vi "RWNoise-Averager.vi"(0 "RW Noise Params":T28, 5 "Runtime":T2={"Stimulus"={"Waveform"={"Type"=enum."Tone", "Tone"={"Frequency (kHz)"=0.0, "Last Freq"=0.0, "Last Phase"=0.0}, "Pulse Train"={"Pulse width (us)"=0.0, "Pulse rate (Hz)"=0.0, "Gap (ms)"=0.0, "Polarity"=enum."POS", "PT State"={"Template"=[], "Nperiod"=0, "Index"=0, "Pulse Rate (Hz)"=0.0, "Phase (cycles)"=0.0, "Noff"=0}, "Asynch"=FALSE}, "Noise"={"InvFilt"=FALSE, "Noise"=[], "CurPt"=0, "Aweight"=FALSE, "Seed"=0, "afile"=path ""}, "File"={"Filename"=path "", "Signal"=[], "Channel"=0, "stream"=FALSE, "offset"=0, "nreps"=0, "loops"=0, "Randomize"=FALSE, "order"=[], "Seed"=0, "Tokens"=0}, "FMSweep"={"Rate (oct/s)"=0.0, "Fmin (Hz)"=0.0, "Fmax (Hz)"=0.0, "Ramp (ms)"=0.0, "Linear"=FALSE}, "Chirp Train"={"Params"={"Fmin (kHz)"=4.0, "Fmax (kHz)"=64.0, "Compensate"=FALSE, "Duration (ms)"=2.0}, "Data"={"WF"=[]}}, "Complex Tone"={"Params"={"F0 (Hz)"=0.0, "Band"={"Flow (Hz)"=0.0, "Fhigh (Hz)"=0.0}, "Phase"=enum."Cosine", "Min F0 (Hz)"=0.0, "Max F0 (Hz)"=0.0, "ContinRandPhase"=FALSE, "Max peak factor"=inf, "Max mod depth"=2.0, "MinHarmNum"=0, "MaxHarmNum"=0, "Level Mode"=enum."per component", "% jitter"=0.0}, "Data"={"Ncomp"=0, "MinHarm"=0, "Phase"=[], "Amplitude"=[], "Npts/frame"=0, "Last F0"=0.0, "Fmin"=0.0, "Fmax"=0.0, "Lslope"=0.0, "randphase"=FALSE, "overall rms"=FALSE, "fmult"=[], "jittered"=FALSE}}, "Moving Ripple"={"Params"={"Fmin"=0.0, "Fmax"=0.0, "Density"=0.0, "Velocity"=0.0, "Depth"=0.0, "Phase"=0.0, "Comp/oct"=0}, "Data"={"Freq"=[], "A"=[], "phase"=[], "Phase"=0.0}}}, "Filter"={"Type"=enum."Lowpass", "CF (kHz)"=0.0, "BW (kHz)"=0.0, "Cascade"=FALSE, "Quadrature"=FALSE, "Scale Factor"=0.0, "Stages"=[], "Class"=enum."Elliptic", "Order"=0, "BWUnits"=enum."Linear"}, "Burst"={"Active"=FALSE, "Delay (ms)"=0.0, "Duration (ms)"=0.0, "Ramp (ms)"=0.0, "Rate (Hz)"=0.0, "Trepeat (ms)"=0.0, "Repeat"=FALSE}, "Level"={"Level"=0.0, "Units"=enum."dB atten", "Max"=0.0, "Multiplier"=0.0, "Cal File"=path "", "Cal"={"Freq (Hz)"=[], "Mag (dB SPL)"=[], "Phase (deg)"=[]}}, "Name"="", "Advanced"={"Rep Mask"="", "AltPol"=FALSE, "Var"="", "Expr"="", "Persist"=FALSE}, "SAM"={"Active"=FALSE, "Frequency (Hz)"=0.0, "Depth"=0.0, "Init Phase (cycles)"=0.0, "phase (degrees)"=0.0, "Asynch"=FALSE}}, "Fs (Hz)"=0.0, "AO Npts"=0, "AO Channels"=[], "Active"=FALSE, "AINpts"=0, "WinPts"=0, "NUpdate"=0} {"Stimulus"."Filter"."Stages"."IIR Filter"."Forward Coefficients" format="%.4f"; "Stimulus"."Filter"."Stages"."IIR Filter"."Reverse Coefficients" format="%.4f"}, 11 "error in (no error)":errorcluster, 12 "Refs":T1) -> (8 "Spectrum (uV)":dbl[](array[numeric]), 15 "error out":errorcluster)   [LabVIEW 2020]
uses:
  RWNoise Params.ctl
  epl-vi-lib/Utility VIs/Type Defs/Left-Right ring.ctl
  RWNoise-Runtime Data.ctl
  epl-vi-lib/Signal Synthesis VIs/Controls/Stimulus Channel (Full)/Full Stimulus Channel Data.ctl
  epl-vi-lib/Signal Synthesis VIs/Controls/Waveform XCtl/Waveform Data.ctl
  epl-vi-lib/Signal Synthesis VIs/Controls/Waveform XCtl/Waveform Enum.ctl
  epl-vi-lib/Signal Synthesis VIs/Waveform VIs/Tone VIs/Tone Params.ctl
  epl-vi-lib/Signal Synthesis VIs/Waveform VIs/Pulse Train VIs/Pulse Train Params.ctl
  epl-vi-lib/Signal Synthesis VIs/Waveform VIs/Pulse Train VIs/Pulse Polarity.ctl
  epl-vi-lib/Signal Synthesis VIs/Waveform VIs/Pulse Train VIs/PT-Continuous State.ctl
  epl-vi-lib/Signal Synthesis VIs/Waveform VIs/Noise VIs/Noise Params.ctl
  epl-vi-lib/Signal Synthesis VIs/Waveform VIs/File VIs/StimFile-Params.ctl
  epl-vi-lib/Signal Synthesis VIs/Waveform VIs/FM Sweep VIs/FM Sweep Params.ctl
  epl-vi-lib/Signal Synthesis VIs/Waveform VIs/Chirp Train VIs/Chirp Train.ctl
  epl-vi-lib/Signal Synthesis VIs/Waveform VIs/Chirp Train VIs/Chirp Train Params.ctl
  epl-vi-lib/Signal Synthesis VIs/Waveform VIs/Complex Tone VIs/CT-Params.ctl
  epl-vi-lib/Signal Synthesis VIs/Waveform VIs/Complex Tone VIs/CT-Phase Enum.ctl
  epl-vi-lib/Signal Synthesis VIs/Waveform VIs/Complex Tone VIs/CT-Runtime Data.ctl
  epl-vi-lib/Signal Synthesis VIs/Waveform VIs/Moving Ripple VIs/Moving Ripple.ctl
  epl-vi-lib/Signal Synthesis VIs/Waveform VIs/Moving Ripple VIs/Moving Ripple.Params.ctl
  epl-vi-lib/Signal Synthesis VIs/Waveform VIs/Moving Ripple VIs/Moving Ripple.Data.ctl
  epl-vi-lib/Signal Synthesis VIs/Controls/Advanced Filter XCtl/Filter Data.ctl
  epl-vi-lib/Signal Synthesis VIs/Filter VIs/Filter-Bandwidth Units.ctl
  epl-vi-lib/Signal Synthesis VIs/Controls/Burst XCtl/Burst Data.ctl
  epl-vi-lib/Signal Synthesis VIs/Controls/Level XCtl/Level Data.ctl
  epl-vi-lib/Signal Synthesis VIs/Controls/Level XCtl/Level Units.ctl
  epl-vi-lib/Signal Synthesis VIs/Controls/Advanced Options XCtl/Advanced Stimulus Options.ctl
  epl-vi-lib/Signal Synthesis VIs/Modulation VIs/SAM VIs/SAM Params.ctl
  RWNoise-Control Refs.ctl
  <vilib>/Analysis/4window.llb/Hanning Window (DBL).vi
  <vilib>/Analysis/4window.llb/AllCosWindow (DBL).vi
  <vilib>/Analysis/NI_AALPro.lvlib
  epl-vi-lib/Signal Synthesis VIs/Controls/Advanced Filter XCtl/Advanced Filter XCtl.xctl
  epl-vi-lib/Signal Synthesis VIs/Controls/Level XCtl/Level XCtl.xctl
  epl-vi-lib/Signal Synthesis VIs/Controls/Burst XCtl/Burst Control.xctl
  epl-vi-lib/Signal Synthesis VIs/Controls/Waveform XCtl/Waveform XCtl.xctl
  epl-vi-lib/Signal Synthesis VIs/Controls/Advanced Options XCtl/Advanced Stimulus Options.xctl
  epl-vi-lib/Signal Synthesis VIs/Controls/Stimulus Channel (Full)/Stimulus Channel (Full).xctl
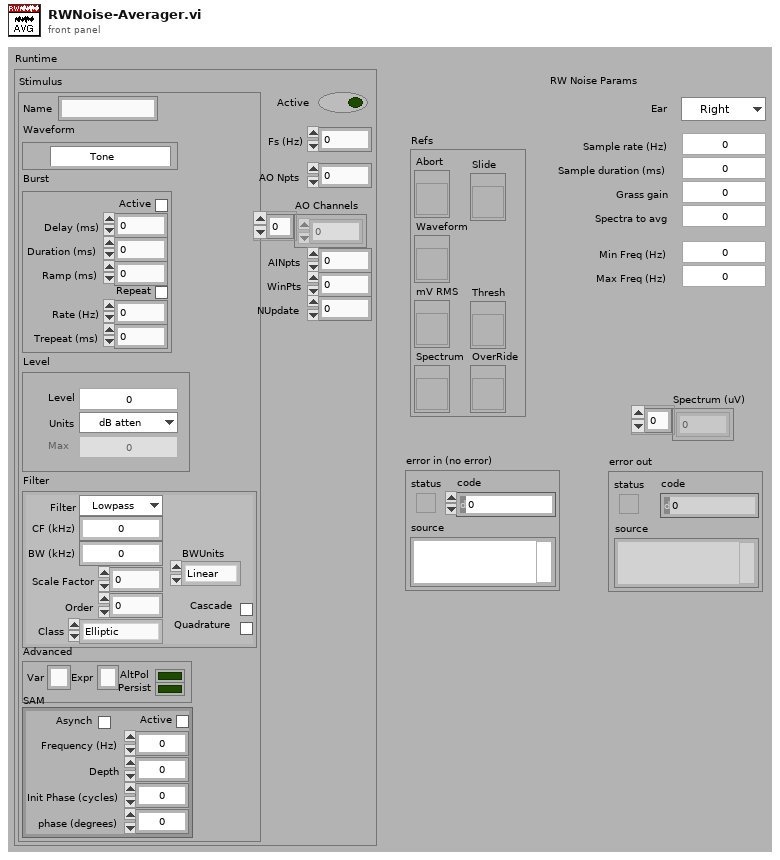
[diagram p1: front panel]
types:
  T1 = typedef "RWNoise-Control Refs.ctl" = cluster{"Abort":refnum<vi>, "Waveform":refnum<vi>, "mV RMS":refnum<vi>, "Spectrum":refnum<vi>, "Slide":refnum<vi>, "Thresh ":refnum<vi>, "OverRide":refnum<vi>}
  T2 = typedef "RWNoise-Runtime Data.ctl" = cluster{"Stimulus":T3, "Fs (Hz)":dbl, "AO Npts":i32, "AO Channels":i32[], "Active":bool, "AINpts":i32, "WinPts":i32, "NUpdate":i32}
  T3 = typedef "Stimulus Channel (Full).xctl/Full Stimulus Channel Data.ctl" = cluster{"Waveform":T4, "Filter":T21, "Burst":T23, "Level":T24, "Name":string, "Advanced":T26, "SAM":T27}
  T4 = typedef "Waveform XCtl.xctl/Waveform Data.ctl" = cluster{"Type":T5, "Tone":T6, "Pulse Train":T7, "Noise":T10, "File":T11, "FMSweep":T12, "Chirp Train":T13, "Complex Tone":cluster{"Params":T15, "Data":T17}, "Moving Ripple":T18}
  T5 = typedef "Waveform Enum.ctl" = enum16{"OFF", "Tone", "Noise", "Pulse Train", "File", "FM Sweep", "Chirp Train", "Complex Tone", "FM Tone", "Moving Ripple"}
  T6 = typedef "Tone Params.ctl" = cluster{"Frequency (kHz)":dbl, "Last Freq":dbl, "Last Phase":dbl}
  T7 = typedef "Pulse Train Params.ctl" = cluster{"Pulse width (us)":dbl, "Pulse rate (Hz)":dbl, "Gap (ms)":dbl, "Polarity":T8, "PT State":T9, "Asynch":bool}
  T8 = typedef "Pulse Polarity.ctl" = enum16{"POS", "NEG", "POS-NEG", "NEG-POS"}
  T9 = typedef "PT-Continuous State.ctl" = cluster{"Template":dbl[], "Nperiod":i32, "Index":i32, "Pulse Rate (Hz)":dbl, "Phase (cycles)":dbl, "Noff":i32}
  T10 = typedef "Noise Params.ctl" = cluster{"InvFilt":bool, "Noise":dbl[], "CurPt":i32, "Aweight":bool, "Seed":i32, "afile":path}
  T11 = typedef "StimFile-Params.ctl" = cluster{"Filename":path, "Signal":dbl[], "Channel":i32, "stream":bool, "offset":i32, "nreps":i32, "loops":i32, "Randomize":bool, "order":i32[], "Seed":i32, "Tokens":i32}
  T12 = typedef "FM Sweep Params.ctl" = cluster{"Rate (oct/s)":dbl, "Fmin (Hz)":dbl, "Fmax (Hz)":dbl, "Ramp (ms)":dbl, "Linear":bool}
  T13 = typedef "Chirp Train.ctl" = cluster{"Params":T14, "Data":cluster{"WF":dbl[]}}
  T14 = typedef "Chirp Train Params.ctl" = cluster{"Fmin (kHz)":dbl, "Fmax (kHz)":dbl, "Compensate":bool, "Duration (ms)":dbl}
  T15 = typedef "CT-Params.ctl" = cluster{"F0 (Hz)":dbl, "Band":cluster{"Flow (Hz)":dbl, "Fhigh (Hz)":dbl}, "Phase":T16, "Min F0 (Hz)":dbl, "Max F0 (Hz)":dbl, "ContinRandPhase":bool, "Max peak factor":dbl, "Max mod depth":dbl, "MinHarmNum":i32, "MaxHarmNum":i32, "Level Mode":enum16{"per component", "overall rms"}, "% jitter":dbl}
  T16 = typedef "CT-Phase Enum.ctl" = enum16{"Cosine", "Random", "Alternating"}
  T17 = typedef "CT-Runtime Data.ctl" = cluster{"Ncomp":i32, "MinHarm":i32, "Phase":dbl[], "Amplitude":dbl[], "Npts/frame":i32, "Last F0":dbl, "Fmin":dbl, "Fmax":dbl, "Lslope":dbl, "randphase":bool, "overall rms":bool, "fmult":dbl[], "jittered":bool}
  T18 = typedef "Moving Ripple.ctl" = cluster{"Params":T19, "Data":T20}
  T19 = typedef "Moving Ripple.Params.ctl" = cluster{"Fmin":dbl, "Fmax":dbl, "Density":dbl, "Velocity":dbl, "Depth":dbl, "Phase":dbl, "Comp/oct":i32}
  T20 = typedef "Moving Ripple.Data.ctl" = cluster{"Freq":dbl[], "A":dbl[], "phase":dbl[], "Phase":dbl}
  T21 = typedef "Advanced Filter XCtl.xctl/Filter Data.ctl" = cluster{"Type":enum16{"Lowpass", "Highpass", "Bandpass", "Bandstop", "OFF"}, "CF (kHz)":dbl, "BW (kHz)":dbl, "Cascade":bool, "Quadrature":bool, "Scale Factor":dbl, "Stages":cluster{"IIR Filter":cluster{"filter structure":enum32{"IIR 2nd Order", "IIR 4th Order"}, "Reverse Coefficients":dbl[], "Forward Coefficients":dbl[]}, "State":dbl[]}[], "Class":enum16{"Elliptic", "Butterworth"}, "Order":i32, "BWUnits":T22}
  T22 = typedef "Filter-Bandwidth Units.ctl" = enum16{"Linear", "Octaves", "Min-Max"}
  T23 = typedef "Burst Control.xctl/Burst Data.ctl" = cluster{"Active":bool, "Delay (ms)":dbl, "Duration (ms)":dbl, "Ramp (ms)":dbl, "Rate (Hz)":dbl, "Trepeat (ms)":dbl, "Repeat":bool}
  T24 = typedef "Level XCtl.xctl/Level Data.ctl" = cluster{"Level":dbl, "Units":T25, "Max":dbl, "Multiplier":dbl, "Cal File":path, "Cal":cluster{"Freq (Hz)":dbl[], "Mag (dB SPL)":dbl[], "Phase (deg)":dbl[]}}
  T25 = typedef "Level Units.ctl" = enum16{"dB atten", "dB SPL", "dB re 1 Vrms", "dB V/Hz½", "mW", "dB HL", "Volts", "dB mW"}
  T26 = typedef "Advanced Stimulus Options.xctl/Advanced Stimulus Options.ctl" = cluster{"Rep Mask":string, "AltPol":bool, "Var":string, "Expr":string, "Persist":bool}
  T27 = typedef "SAM Params.ctl" = cluster{"Active":bool, "Frequency (Hz)":dbl, "Depth":dbl, "Init Phase (cycles)":dbl, "phase (degrees)":dbl, "Asynch":bool}
  T28 = typedef "RWNoise Params.ctl" = cluster{"Sample rate (Hz)":dbl, "Sample duration (ms)":dbl, "Grass gain":dbl, "Min Freq (Hz)":dbl, "Max Freq (Hz)":dbl, "Spectra to avg":i32, "Ear":T29}
  T29 = typedef "Left-Right ring.ctl" = enum16{"Right", "Left"}
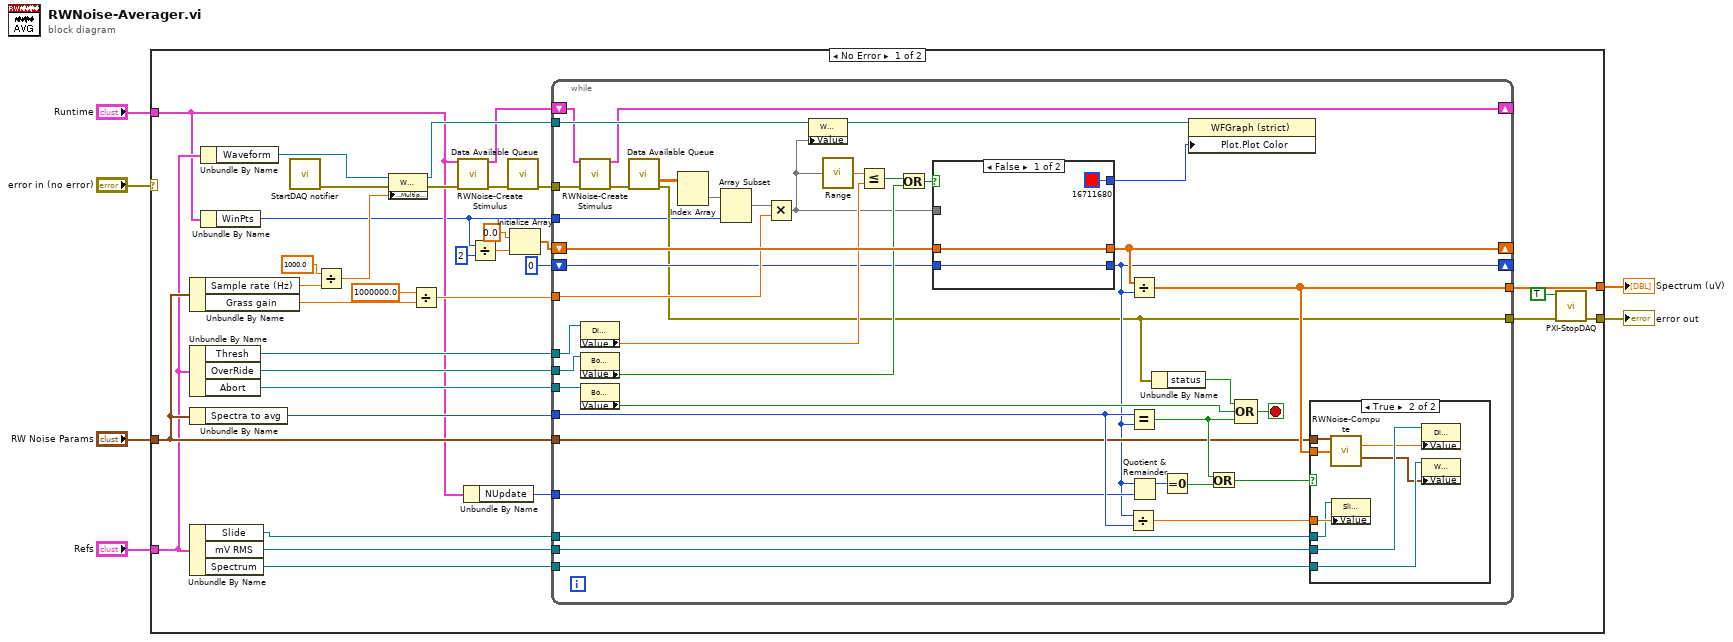
[diagram p0: block diagram]
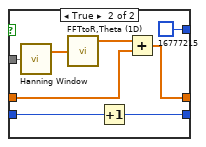
[diagram p2: hidden frame]
diagram:
  n1 = case shown="No Error" "error in (no error)" {
    selector: "error in (no error)" -> [_ w101]
    tunnel: "RW Noise Params" -> [w21 _]
    tunnel: [w30 w101] -> w4
    tunnel: [w23 _] -> w3
    tunnel: "Runtime" -> [w8 _]
    tunnel: "Refs" -> [w19 _]
    frame No Error {
      n2 = Unbundle By Name(w21) -> ("Sample rate (Hz)"=w38:dbl, "Grass gain"=w40:dbl)
      n3 = Unbundle By Name(w19) -> ("Thresh"=w14:refnum<vi>, "OverRide"=w13:refnum<vi>, "Abort"=w24:refnum<vi>)
      n4 = Unbundle By Name(w21) -> ("Spectra to avg"=w20:i32)
      n5 = Unbundle By Name(w19) -> ("Slide"=w18:refnum<vi>, "mV RMS"=w17:refnum<vi>, "Spectrum"=w16:refnum<vi>)
      n6 = Unbundle By Name(w19) -> ("Waveform"=w25:refnum<vi>)
      n7 = Unbundle By Name(w8) -> ("WinPts"=w7:i32)
      n8 = call "StartDAQ notifier.vi"() -> ("error out"=w31:errorcluster)  [unwired: 7 in]
      n9 = Divide(x=1000.0, y=w38) -> (x/y=w35:dbl)
      n10 = property class="WFGraph (strict)"(reference=w25, error in=w31, "XScale.Multiplier"=w35) -> (reference out=w34:refnum<vi>, error out=w36:errorcluster)
      n11 = Divide(x=1000000.0, y=w40) -> (x/y=w33:dbl)
      n12 = call "RWNoise-Create Stimulus.vi"("Runtime"=w8, "error in (no error)"=w36) -> ("Runtime Out"=w26:T2, "error out"=w27:errorcluster)  [unwired: 12 in]
      n13 = Unbundle By Name(w8) -> ("NUpdate"=w22:i32)
      n14 = Divide(x=w7, y=2) -> (x/y=w11:dbl)
      n15 = call "Data Available Queue.vi"("error in (no error)"=w27) -> ("error out"=w28:errorcluster)  [unwired: 10 in, 4 out]
      n16 = Initialize Array(0.0 ("element"), w11) -> (w9:dbl[])
      n17 = while {
        tunnel: w28 -> [w81]
        shift-right: [w68] -> _
        shift-left: w9 -> [w78]
        tunnel: w33 -> [w77]
        tunnel: w20 -> [w67]
        tunnel: [w44] -> w39
        tunnel: w34 -> [w74]
        shift-right: [w70] -> _
        shift-left: w26 -> [w71]
        tunnel: w24 -> [w69]
        tunnel: [w61] -> w23
        tunnel: w22 -> [w66]
        tunnel: w21 -> [w60]
        tunnel: w18 -> [w58]
        tunnel: w17 -> [w57]
        tunnel: w16 -> [w56]
        shift-right: [w45] -> _
        shift-left: 0 -> [w46]
        tunnel: w14 -> [w54]
        tunnel: w13 -> [w53]
        tunnel: w7 -> [w43]
        stop <- w75 stop-if-true
        n18 = call "RWNoise-Create Stimulus.vi"("Runtime"=w71, "error in (no error)"=w81) -> ("Runtime Out"=w70:T2, "error out"=w72:errorcluster)  [unwired: 12 in]
        n19 = property class="DigNum (strict)"(reference=w54) -> ("Value"=w51:dbl)  [unwired: 1 in, 2 out]
        n20 = property class="Bool (strict)"(reference=w53) -> ("Value"=w49:bool)  [unwired: 1 in, 2 out]
        n21 = property class="Bool (strict)"(reference=w69) -> ("Value"=w73:bool)  [unwired: 1 in, 2 out]
        n22 = call "Data Available Queue.vi"("error in (no error)"=w72) -> ("AI Waveforms"=w80:dbl[][], "error out"=w44:errorcluster)  [unwired: 10 in, 3 out]
        n23 = Index Array(array=w80) -> (element=w79:dbl[])  [unwired: 2 in]
        n24 = Array Subset(array=w79, length=w43) -> (w55:dbl[])  [unwired: 1 in]
        n25 = Multiply(x=w55, y=w77) -> (x*y=w47:dbl[])
        n26 = property class="WFGraph (strict)"(reference=w74, "Value"=w47) -> (reference out=w42:refnum<vi>)  [unwired: 1 in, 1 out]
        n27 = call "Range.vi"("Array"=w47) -> ("Range"=w52:dbl)
        n28 = Less Or Equal?(x=w52, y=w51) -> (x <= y?=w50:bool)
        n29 = Or(x=w50, y=w49) -> (x .or. y?=w48:bool)
        n30 = case shown="False" w48 {
          tunnel: w78 -> [w84 w91]
          tunnel: [w84 w90] -> w68
          tunnel: w47 -> [_ w88]
          tunnel: w46 -> [w83 w87]
          tunnel: [w83 w86] -> w45
          tunnel: [u32 16711680 u32 16777215] -> w41
          frame False {
          }
          frame True {
            n31 = call-poly <vilib>:"Hanning Window.vi"("X"=w88) -> ("Windowed X"=w89:dbl[])  [unwired: 1 out]
            n32 = call "FFTtoR,Theta (1D).VI"("X"=w89) -> ("+Freq. Mag of FFT"=w92:dbl[])  [unwired: 1 in, 1 out]
            n33 = Increment(x=w87) -> (x+1=w86:i32)
            n34 = Add(x=w92, y=w91) -> (x+y=w90:dbl[])
          }
        }
        n35 = Divide(x=w45, y=w67) -> (x/y=w59:dbl)
        n36 = Divide(x=w68, y=w45) -> (x/y=w61:dbl[])
        n37 = Equal?(x=w67, y=w45) -> (x = y?=w65:bool)
        n38 = Quotient & Remainder(x=w45, y=w66) -> (x-y*floor(x/y)=w64:i32)  [unwired: 1 out]
        n39 = Unbundle By Name(w44) -> ("status"=w76:bool)
        n40 = Equal To 0?(x=w64) -> (x = 0?=w63:bool)
        n41 = property class="WFGraph (strict)"(reference=w42, "Plot.Plot Color"=w41) -> ()  [unwired: 1 in, 2 out]
        n42 = Or(x=w65, y=w63) -> (x .or. y?=w62:bool)
        n43 = Compound Arithmetic op=OR(w76, w73, w65) -> (w75:bool)
        n44 = case shown="True" w62 {
          tunnel: w61 -> [_ w100]
          tunnel: w60 -> [_ w99]
          tunnel: w59 -> [_ w98]
          tunnel: w58 -> [_ w97]
          tunnel: w57 -> [_ w96]
          tunnel: w56 -> [_ w94]
          frame False {
          }
          frame True {
            n45 = call "RWNoise-Compute.vi"("RW Noise Params"=w99, "Spectrum (uV)"=w100) -> ("RW Noise (uV)"=w95:dbl, "Spectrum (uV/sqrt(Hz))"=w93:waveform(dbl))  [unwired: 11 in, 1 out]
            n46 = property class="Slide (strict)"(reference=w97, "Value"=w98) -> ()  [unwired: 1 in, 2 out]
            n47 = property class="DigNum (strict)"(reference=w96, "Value"=w95) -> ()  [unwired: 1 in, 2 out]
            n48 = property class="WFGraph (strict)"(reference=w94, "Value"=w93) -> ()  [unwired: 1 in, 2 out]
          }
        }
      }
      n49 = call "PXI-StopDAQ.vi"("error in (no error)"=w39, "Wait for DAQ to stop? (T)"=TRUE ("Wait for DAQ to stop?")) -> ("error out"=w30:errorcluster)  [unwired: 5 in]
    }
    frame Error {
    }
  }
  "error out" <- w4
  "Spectrum (uV)" <- w3
